vi "Ping.vi"(0 "WebSocket Connection in":refnum<k5>, 1 "timeout ms (5000)":i32=5000, 9 "Data":string, 11 "error in (no error)":errorcluster, 12 "Mask payload?":bool) -> (4 "WebSocket Connection in":refnum<k5>, 15 "error out":errorcluster)   [LabVIEW 2021, in "LV WebSockets.lvlib"]
doc: "Sends the ping frame to the Websocket."
uses:
  LV WebSockets.lvlib
  Opcode.ctl
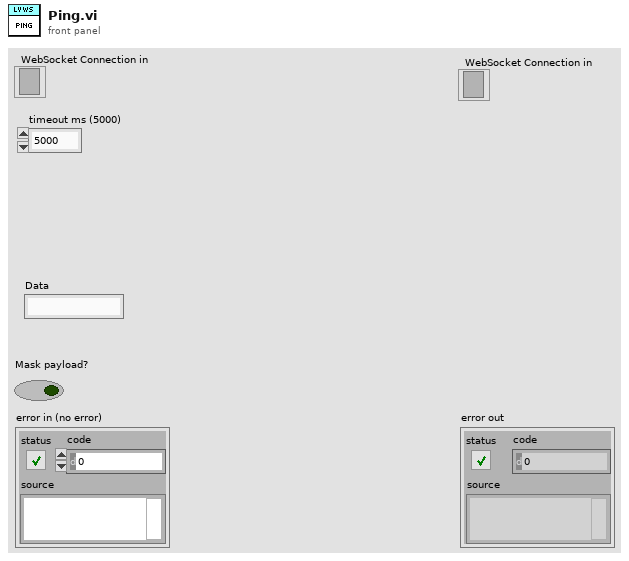
[diagram p1: front panel]
types:
  T1 = typedef "LV WebSockets.lvlib/Opcode.ctl" = enum8{"Continuation Frame", "Text Frame", "Binary Frame", "Reserved 3", "Reserved 4", "Reserved 5", "Reserved 6", "Reserved 7", "Connection Close", "Ping", "Pong", "Reserved B", "Reserved C", "Reserved D", "Reserved F"}
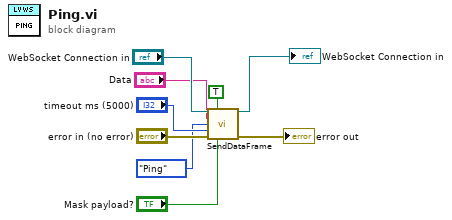
[diagram p0: block diagram]
diagram:
  n1 = call "SendDataFrame.vi"("WebSocket Connection in"="WebSocket Connection in", "Final Frame Bit  (F)"=TRUE ("FIN Bit (F)"), "Data"="Data", "Opcode"=Opcode."Ping", "timeout ms (5000)"="timeout ms (5000)", "error in (no error)"="error in (no error)", "Mask payload?"="Mask payload?") -> ("WebSocket Connection out"=→"WebSocket Connection in":refnum<k5>, "error out"=→"error out":errorcluster)  [unwired: 7 in]
